vi "TTTRHDR_P_write.vi"(8 "error in (no error)":errorcluster, 10 "TTTRHDR_P":T1, 11 "refnum in":refnum<file>) -> (0 "error out":errorcluster, 3 "refnum out":refnum<file>)   [LabVIEW 2012]
uses:
  TTTR_data_headers/TTTRHDR_P.ctl
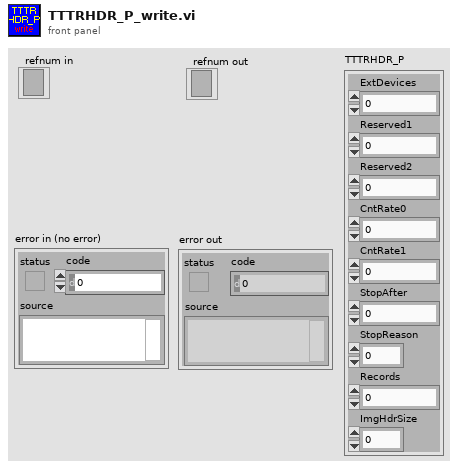
[diagram p1: front panel]
types:
  T1 = typedef "TTTRHDR_P.ctl" = cluster{"ExtDevices":i32, "Reserved1":i32, "Reserved2":i32, "CntRate0":i32, "CntRate1":i32, "StopAfter":i32, "StopReason":i32, "Records":u32, "ImgHdrSize":i32}
  T2 = enum16{"big-endian, network order", "native, host order", "little-endian"}
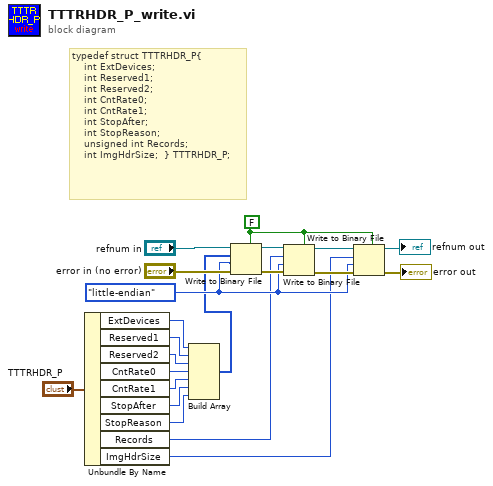
[diagram p0: block diagram]
diagram:
  w3 = FALSE ("prepend array or string size? (T)")
  w13 = T2."little-endian" ("byte order (0:big-endian, network order)")
  # "typedef struct TTTRHDR_P{\n\t\t\t\tint ExtDevices;\n\t\t\t\tint Reserved1;\n\t\t\t\tint Reserved2;\t\t\t\n\t\t\t\tint CntRate0;\n\t\t\t\tint CntRate1;\n\t\t\t\tint StopAfter;\n\t\t\t\tint StopReason;\n\t\t\t\tunsigned int Records;\n\t\t\t\tint ImgHdrSize;\t\t} TTTRHDR_P;"
  n1 = Unbundle By Name("TTTRHDR_P") -> ("ExtDevices"=w11:i32, "Reserved1"=w10:i32, "Reserved2"=w9:i32, "CntRate0"=w8:i32, "CntRate1"=w7:i32, "StopAfter"=w6:i32, "StopReason"=w5:i32, "Records"=w2:u32, "ImgHdrSize"=w1:i32)
  n2 = Build Array(w11, w10, w9, w8, w7, w6, w5) -> (w4:i32[])
  n3 = Write to Binary File(file (use dialog)="refnum in", data=w4, error in="error in (no error)", 5:w3, 9:w13) -> (refnum out=w20:refnum<file>, error out=w21:errorcluster)  [unwired: 1 in, 1 out]
  n4 = Write to Binary File(file (use dialog)=w20, data=w2, error in=w21, 5:w3, 9:w13) -> (refnum out=w15:refnum<file>, error out=w17:errorcluster)  [unwired: 1 in, 1 out]
  n5 = Write to Binary File(file (use dialog)=w15, data=w1, error in=w17, 5:w3, 9:w13) -> (refnum out=→"refnum out":refnum<file>, error out=→"error out":errorcluster)  [unwired: 1 in, 1 out]
